vi "Create Sense Reference Control.vi"(8 "error in (no error)":errorcluster, 11 "Device Item Ref in":T1 format="%.0x") -> (0 "error out":errorcluster)   [LabVIEW 2020, in "G5 Regatron Custom Device System Explorer.lvlib"]
uses:
  G5 Regatron Custom Device System Explorer.lvlib
  <vilib>/NI VeriStand/Custom Device API/Custom Device Item Ref.ctl
  <vilib>/NI VeriStand/Custom Device API/Custom Device Channel.ctl
  <vilib>/NI VeriStand/Custom Device API/Custom Device Channel Type.ctl
  <vilib>/NI VeriStand/Custom Device API/Custom Device API.lvlib
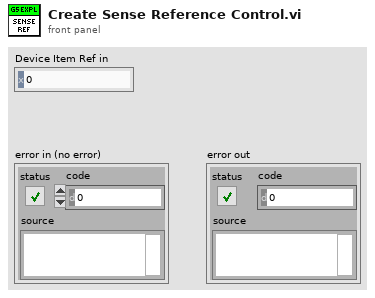
[diagram p1: front panel]
types:
  T1 = typedef "Custom Device API.lvlib/Custom Device Item Ref.ctl" = u64
  T2 = typedef "Custom Device API.lvlib/Custom Device Channel.ctl" = cluster{"Type":T3, "Units":string, "Default Value":dbl, "Faultable":bool, "Scalable":bool}
  T3 = typedef "Custom Device API.lvlib/Custom Device Channel Type.ctl" = enum16{"Input", "Output"}
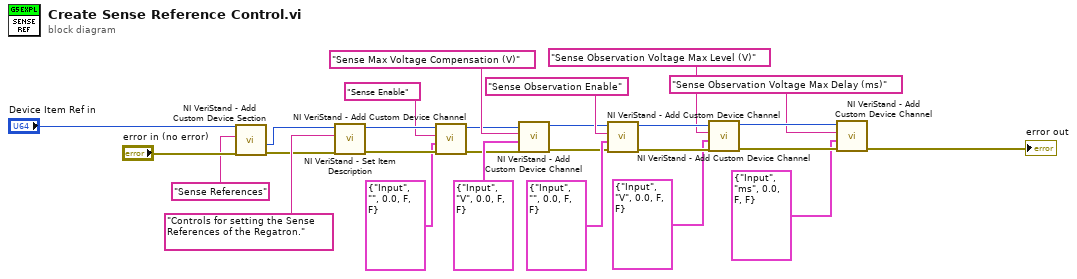
[diagram p0: block diagram]
diagram:
  n1 = call <vilib>:"NI VeriStand - Add Custom Device Section.vi"("error in (no error)"="error in (no error)", "Section Name"="Sense References", "Parent Ref in"="Device Item Ref in") -> ("error out"=w23:errorcluster, "Section Ptr"=w24:T1)  [unwired: 5 in, 2 out]
  n2 = call <vilib>:"NI VeriStand - Set Item Description.vi"("error in (no error)"=w23, "Description"="Controls for setting the Sense References of the Regatron.", "Item Ref in"=w24) -> ("error out"=w26:errorcluster, "Item Ref out"=w25:T1)  [unwired: 6 in, 1 out]
  n3 = call <vilib>:"NI VeriStand - Add Custom Device Channel.vi"("error in (no error)"=w26, "Channel"=T2 {"Type"=enum."Input", "Units"="", "Default Value"=0.0, "Faultable"=FALSE, "Scalable"=FALSE}, "Channel Name"="Sense Enable", "Parent Ref in"=w25) -> ("error out"=w4:errorcluster, "Parent Ref out"=w5:T1)  [unwired: 4 in, 2 out]
  n4 = call <vilib>:"NI VeriStand - Add Custom Device Channel.vi"("error in (no error)"=w4, "Channel"=T2 {"Type"=enum."Input", "Units"="V", "Default Value"=0.0, "Faultable"=FALSE, "Scalable"=FALSE}, "Channel Name"="Sense Max Voltage Compensation (V)", "Parent Ref in"=w5) -> ("error out"=w8:errorcluster, "Parent Ref out"=w9:T1)  [unwired: 4 in, 2 out]
  n5 = call <vilib>:"NI VeriStand - Add Custom Device Channel.vi"("error in (no error)"=w8, "Channel"=T2 {"Type"=enum."Input", "Units"="", "Default Value"=0.0, "Faultable"=FALSE, "Scalable"=FALSE}, "Channel Name"="Sense Observation Enable", "Parent Ref in"=w9) -> ("error out"=w17:errorcluster, "Parent Ref out"=w16:T1)  [unwired: 4 in, 2 out]
  n6 = call <vilib>:"NI VeriStand - Add Custom Device Channel.vi"("error in (no error)"=w17, "Channel"=T2 {"Type"=enum."Input", "Units"="V", "Default Value"=0.0, "Faultable"=FALSE, "Scalable"=FALSE}, "Channel Name"="Sense Observation Voltage Max Level (V)", "Parent Ref in"=w16) -> ("error out"=w19:errorcluster, "Parent Ref out"=w18:T1)  [unwired: 4 in, 2 out]
  n7 = call <vilib>:"NI VeriStand - Add Custom Device Channel.vi"("error in (no error)"=w19, "Channel"=T2 {"Type"=enum."Input", "Units"="ms", "Default Value"=0.0, "Faultable"=FALSE, "Scalable"=FALSE}, "Channel Name"="Sense Observation Voltage Max Delay (ms)", "Parent Ref in"=w18) -> ("error out"=→"error out":errorcluster)  [unwired: 4 in, 3 out]
